vi "toml_to_cluster.vi"(8 "error in (no error)":errorcluster, 11 "toml":string) -> (0 "error out":errorcluster, 3 "tables":variant)   [LabVIEW 2017]
uses:
  toml_token.ctl
  <vilib>/regexp/Match Regular Expression.xnode
panel:
  in  "include comments? (F)":bool
  out "args":string[](array[string])
  out "tokens":T1[](array[typedef])
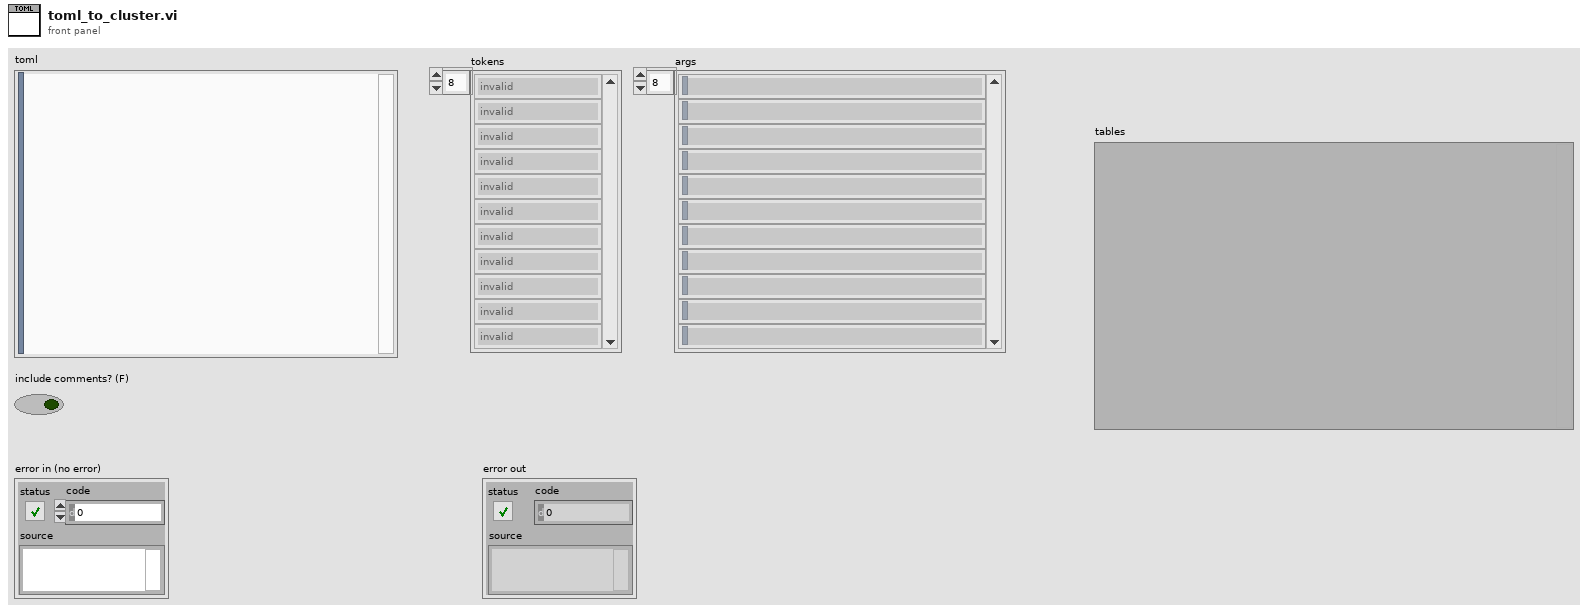
[diagram p1: front panel]
types:
  T1 = typedef "toml_token.ctl" = enum8{"invalid", "bool", "string", "string_start", "int", "uint", "float", "datetime", "array", "inline_table", "table", "table_element", "key", "comment", "comment_inline", "end"}
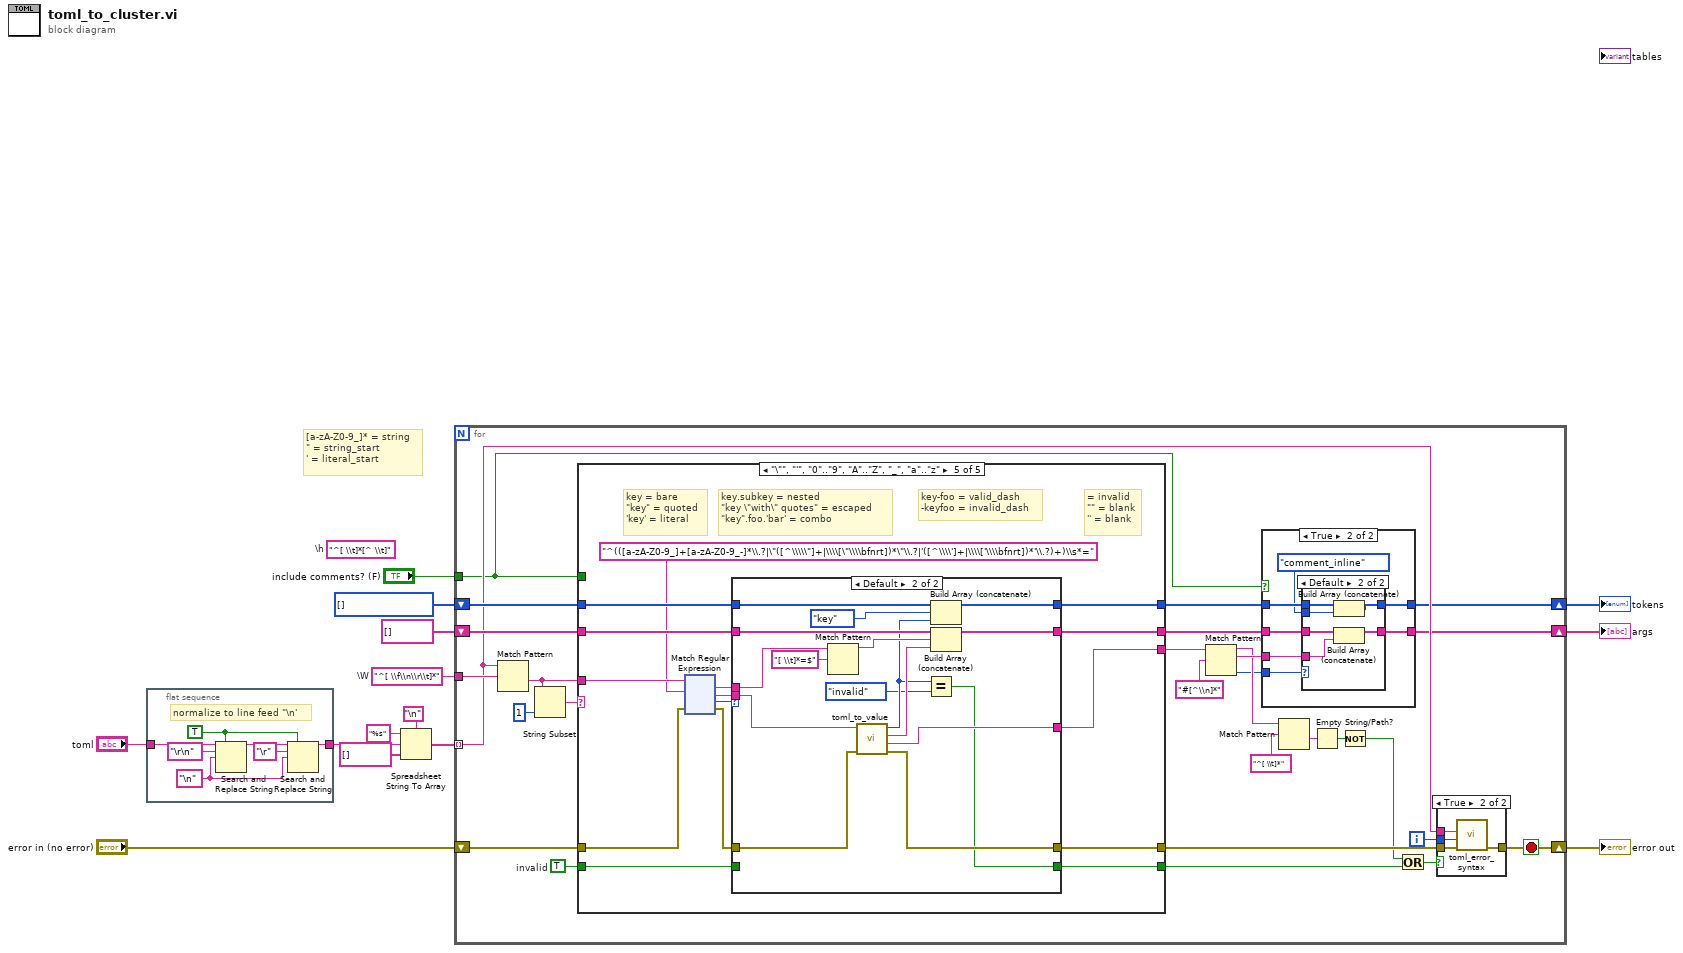
[diagram p0: block diagram]
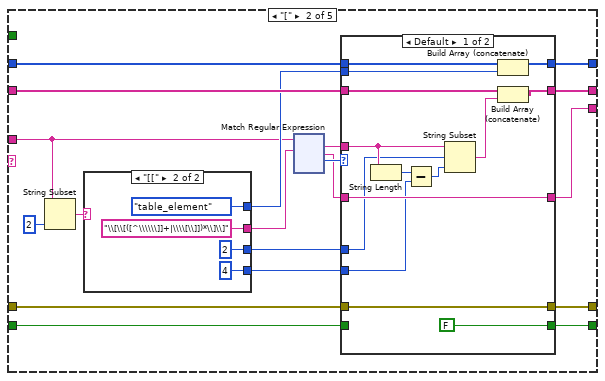
[diagram p5: hidden frame]
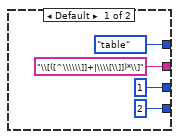
[diagram p6: hidden frame]
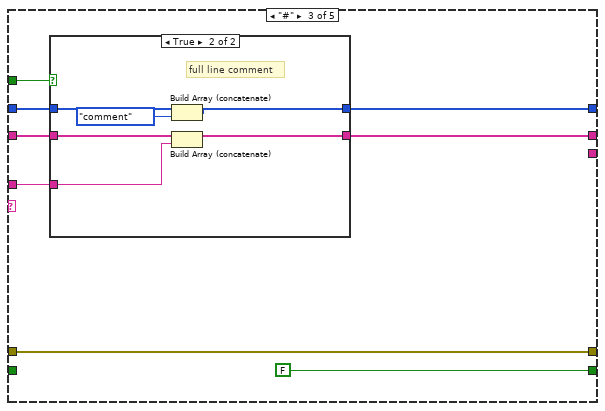
[diagram p8: hidden frame]
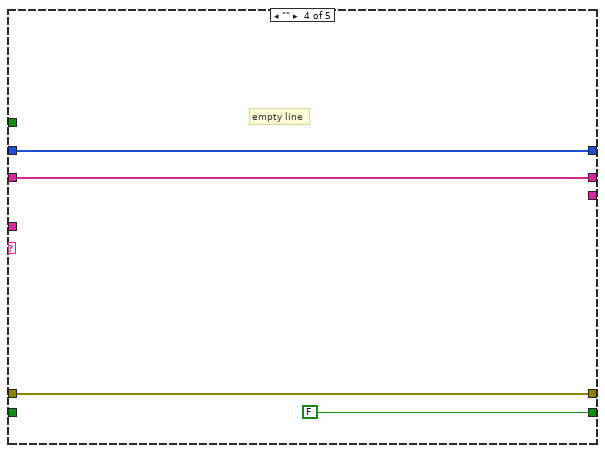
[diagram p10: hidden frame]
diagram:
  w9 = T1[] [] items=["invalid", "bool", "string", "string_start", "int", "uint", "float", "datetime", "array", "inline_table", "table", "table_element", "key", "comment", "comment_inline", "end"]
  w10 = "^[ \\f\\n\\r\\t]*"  # \W
  (unwired) "^[ \\t]*[^ \\t]"  # \h
  # "[a-zA-Z0-9_]* = string\n\" = string_start\n' = literal_start"
  n1 = flat-sequence {
    tunnel: "toml" -> [w16]
    tunnel: [w15] -> w2
    frame #0 {
      w17 = "\n" ("search string")
      w18 = TRUE ("replace all? (F)")
      # "normalize to line feed \"\\n'"
      n2 = Search and Replace String(replace all?=w18, input string=w16, search string="\r\n", replace string=w17) -> (result string=w20:string)  [unwired: 4 in, 3 out]
      n3 = Search and Replace String(replace all?=w18, input string=w20, search string="\r", replace string=w17) -> (result string=w15:string)  [unwired: 4 in, 3 out]
    }
  }
  n4 = Spreadsheet String To Array(delimiter (Tab)="\n", format string="%s", spreadsheet string=w2, array type (2D Dbl)=string[] []) -> (array=w11:string[])
  n5 = for {
    tunnel: w11 -> [w41] mode=indexing
    tunnel: w10 -> [w49]
    shift-right: [w38] -> w5
    shift-left: w9 -> [w47]
    shift-right: [w36] -> w4
    shift-left: string[] [] -> [w46]
    shift-right: [w43] -> w6
    shift-left: "error in (no error)" -> [w45]
    tunnel: "include comments? (F)" -> [w22]
    i -> [w42]
    stop <- w43 stop-if-true
    w40 = TRUE  # invalid
    n6 = Match Pattern(string=w41, regular expression=w49) -> (after substring=w31:string)  [unwired: 1 in, 3 out]
    n7 = String Subset(string=w31, length (rest)=1 ("length (rest)")) -> (substring=w48:string)  [unwired: 1 in]
    n8 = case shown="\"\\\"\", \"'\", \"0\"..\"9\", \"A\"..\"Z\", \"_\", \"a\"..\"z\"" w48 {
      tunnel: [w70 w87 w234 w249 w262] -> w37
      tunnel: w47 -> [w70 w86 w237 w249 w264]
      tunnel: [w69 w85 w235 w248 w261] -> w35
      tunnel: w46 -> [w69 w84 w236 w248 w263]
      tunnel: w31 -> [_ w76 w231 _ w260]
      tunnel: w45 -> [w68 w89 w233 w247 w253]
      tunnel: [w68 w88 w233 w247 w256] -> w44
      tunnel: [w67 w81 FALSE ("invalid") FALSE ("invalid") w255] -> w33
      tunnel: w40 -> [w67 w80 _ _ w254]
      tunnel: [_ w78 _ _ w251] -> w39
      tunnel: w22 -> [_ _ w230 _ _]
      frame Default {
        # "unknown"
      }
      frame "[" {
        n9 = String Subset(string=w76, length (rest)=2 ("length (rest)")) -> (substring=w77:string)  [unwired: 1 in]
        n10 = case shown="\"[[\"" w77 {
          tunnel: [toml_token."table" ("token") toml_token."table_element" ("token")] -> w82
          tunnel: ["\\[([^\\\\\\]]+|\\\\[\\]])*\\]" ("regular expression") "\\[\\[([^\\\\\\]]+|\\\\[\\]])*\\]\\]" ("regular expression")] -> w75
          tunnel: [1 ("x-1") 2 ("x-1")] -> w79
          tunnel: [2 ("x-1") 4 ("x-1")] -> w71
          frame Default {
          }
          frame "[[" {
          }
        }
        n11 = xnode "Match Regular Expression"("input string"=w76, "regular expression"=w75) -> ("whole match"=w73:string, "after match"=w72:string, "offset past match"=w74:i32)  [unwired: 4 in, 2 out]
        n12 = case shown="Default" w74 {
          tunnel: w89 -> [w222 w227]
          tunnel: [w222 w227] -> w88
          tunnel: w73 -> [w225 _]
          tunnel: [w216 w229] -> w87
          tunnel: w86 -> [w224 w229]
          tunnel: [w215 w228] -> w85
          tunnel: w84 -> [w223 w228]
          tunnel: w82 -> [w220 _]
          tunnel: w72 -> [w217 _]
          tunnel: [FALSE ("invalid") w226] -> w81
          tunnel: w80 -> [_ w226]
          tunnel: w79 -> [w212 _]
          tunnel: [w217 _] -> w78
          tunnel: w71 -> [w213 _]
          frame Default {
            n13 = String Length(string=w225) -> (length=w219:i32)
            n14 = Subtract(x=w219, y=w213) -> (x-y=w218:i32)
            n15 = String Subset(string=w225, offset (0)=w212, length (rest)=w218) -> (substring=w221:string)
            n16 = Build Array (concatenate)(w224, w220) -> (w216:T1[])
            n17 = Build Array (concatenate)(w223, w221) -> (w215:string[])
          }
          frame -1 {
          }
        }
      }
      frame "#" {
        n18 = case shown="True" w230 {
          tunnel: w237 -> [w239 w245]
          tunnel: w236 -> [w238 w244]
          tunnel: [w238 w243] -> w235
          tunnel: [w239 w242] -> w234
          tunnel: w231 -> [_ w240]
          frame False {
          }
          frame True {
            # "full line comment"
            n19 = Build Array (concatenate)(w245, toml_token."comment" ("token")) -> (w242:T1[])
            n20 = Build Array (concatenate)(w244, w240) -> (w243:string[])
          }
        }
      }
      frame "" {
        # "empty line"
      }
      frame "\"", "'", "0".."9", "A".."Z", "_", "a".."z" {
        # "key-foo = valid_dash\n-keyfoo = invalid_dash"
        # "= invalid\n\"\" = blank\n'' = blank"
        # "key.subkey = nested\n\"key \\\"with\\\" quotes\" = escaped\n\"key\".foo.'bar' = combo"
        # "key = bare\n\"key\" = quoted\n'key' = literal"
        n21 = xnode "Match Regular Expression"("input string"=w260, "regular expression"="^(([a-zA-Z0-9_]+[a-zA-Z0-9_-]*\\.?|\"([^\\\\\"]+|\\\\[\"\\\\bfnrt])*\"\\.?|'([^\\\\']+|\\\\['\\\\bfnrt])*'\\.?)+)\\s*=" ("key"), "error in"=w253) -> ("whole match"=w257:string, "after match"=w250:string, "offset past match"=w258:i32, "error out"=w252:errorcluster)  [unwired: 3 in, 1 out]
        n22 = case shown="Default" w258 {
          tunnel: w264 -> [w266 w284]
          tunnel: w263 -> [w265 w283]
          tunnel: [w266 w282] -> w262
          tunnel: [w265 w281] -> w261
          tunnel: w257 -> [_ w279]
          tunnel: [w268 w275] -> w256
          tunnel: w252 -> [w268 w276]
          tunnel: [w267 w269] -> w255
          tunnel: w254 -> [w267 _]
          tunnel: [_ w272] -> w251
          tunnel: w250 -> [_ w273]
          frame -1 {
          }
          frame Default {
            n23 = Match Pattern(string=w279, regular expression="[ \\t]*=$") -> (before substring=w278:string)  [unwired: 1 in, 3 out]
            n24 = call "toml_to_value.vi"("error in (no error)"=w276, "toml line"=w273) -> ("error out"=w275:errorcluster, "remaining"=w272:string, "arg"=w274:string, "token"=w271:T1)  [unwired: 6 in]
            n25 = Equal?(x=w271, y=toml_token."invalid") -> (x = y?=w269:bool)
            n26 = Build Array (concatenate)(w284, toml_token."key" ("token"), w271) -> (w282:T1[])
            n27 = Build Array (concatenate)(w283, w278, w274) -> (w281:string[])
          }
        }
      }
    }
    n28 = Match Pattern(string=w39, regular expression="#[^\\n]*") -> (before substring=w26:string, match substring=w28:string, offset past match=w25:i32)  [unwired: 1 in, 1 out]
    n29 = case shown="True" w22 {
      tunnel: [w51 w58] -> w38
      tunnel: w37 -> [w51 w57]
      tunnel: [w50 w56] -> w36
      tunnel: w35 -> [w50 w55]
      tunnel: w28 -> [_ w54]
      tunnel: w25 -> [_ w53]
      frame False {
      }
      frame True {
        n30 = case shown="Default" w53 {
          tunnel: [w60 w66] -> w58
          tunnel: w57 -> [w60 w65]
          tunnel: [w59 w64] -> w56
          tunnel: w55 -> [w59 w63]
          tunnel: w54 -> [_ w62]
          tunnel: toml_token."comment_inline" ("token") -> [_ w61]
          frame -1 {
          }
          frame Default {
            n31 = Build Array (concatenate)(w65, w61) -> (w66:T1[])
            n32 = Build Array (concatenate)(w63, w62) -> (w64:string[])
          }
        }
      }
    }
    n33 = Match Pattern(string=w26, regular expression="^[ \\t]*") -> (after substring=w24:string)  [unwired: 1 in, 3 out]
    n34 = Empty String/Path?(string/path=w24) -> (empty?=w23:bool)
    n35 = Not(x=w23) -> (.not. x?=w34:bool)
    n36 = Or(x=w34, y=w33) -> (x .or. y?=w32:bool)
    n37 = case shown="True" w32 {
      tunnel: w44 -> [w399 w403]
      tunnel: [w399 w402] -> w43
      tunnel: w42 -> [_ w401]
      tunnel: w41 -> [_ w400]
      frame False {
      }
      frame True {
        n38 = call "toml_error_syntax.vi"("error in (no error)"=w403, "line"=w401, "toml"=w400) -> ("error out"=w402:errorcluster)  [unwired: 8 in]
      }
    }
  }
  "error out" <- w6
  "tokens" <- w5
  "args" <- w4
